vi "SG Main.vi"() -> ()   [LabVIEW 2019]
uses:
  UI Controls/redRoundButton.ctl
  TypeDefs/SG States.ctl
  TypeDefs/SG Data.ctl
  Player/Player.lvclass
  Simon_Engine/Simon_Engine.lvclass
  TextDisplay/TextDisplay Class.lvclass
  Messages/simonMessages/simonMessages.lvclass
  uiControlsMgr/uiControlsMgr.lvclass
  Player/Player.lvclass/Player.ctl
  e5cb8d52-8214-47cd-985f-bfccfb8a6597.vi
  <vilib>/ErrorRing/Error Ring.xnode
panel:
  in  "0008":bool caption="REPETE"
  in  "0007":bool caption="MAIS LONGO"
  in  "0006":T1 caption="PARTIDA"
  in  "0005":u8(slide)=1 caption="HABILIDADE" min=1 max=5 step=1 scale=1.0..4.0
  in  "0001":bool caption="Vermelho"
  in  "0004":bool caption="Amarelo"
  in  "0003":bool caption="Verde"
  in  "0002":bool caption="Azul"
  out "0009":string caption="MOSTRADOR"
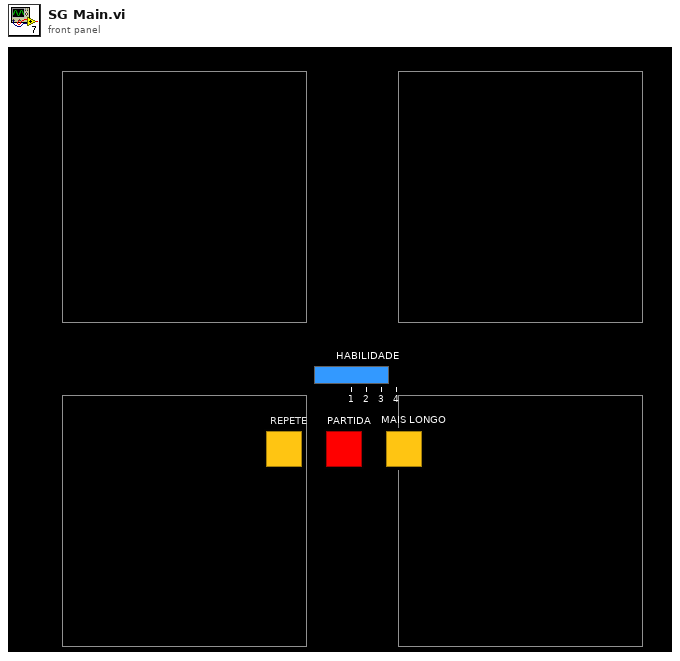
[diagram p1: front panel]
types:
  T1 = typedef "redRoundButton.ctl" = bool
  T2 = typedef "SG Data.ctl" = cluster{"Player":refnum<class "Player.lvclass">, "Engine":refnum<class "Simon_Engine.lvclass">, "TextDisplay":refnum<class "TextDisplay Class.lvclass">, "Messages":refnum<class "simonMessages.lvclass">, "UI Controls Mgr":refnum<class "uiControlsMgr.lvclass">, "High Scores":map{string, i32}, "This VI":refnum<vi>, "LanguageFiles":cluster{"captionsFile":string, "messageFile":string}}
  T3 = typedef "SG States.ctl" = enum16{"Initialize References", "Initialize Classes", "Wait on Event", "Start Game", "Last", "Longest", "Play Game", "Check Move", "Win", "Lost", "HighScores", "Exit"}
  T4 = cluster{"captionsFile":string, "messageFile":string}
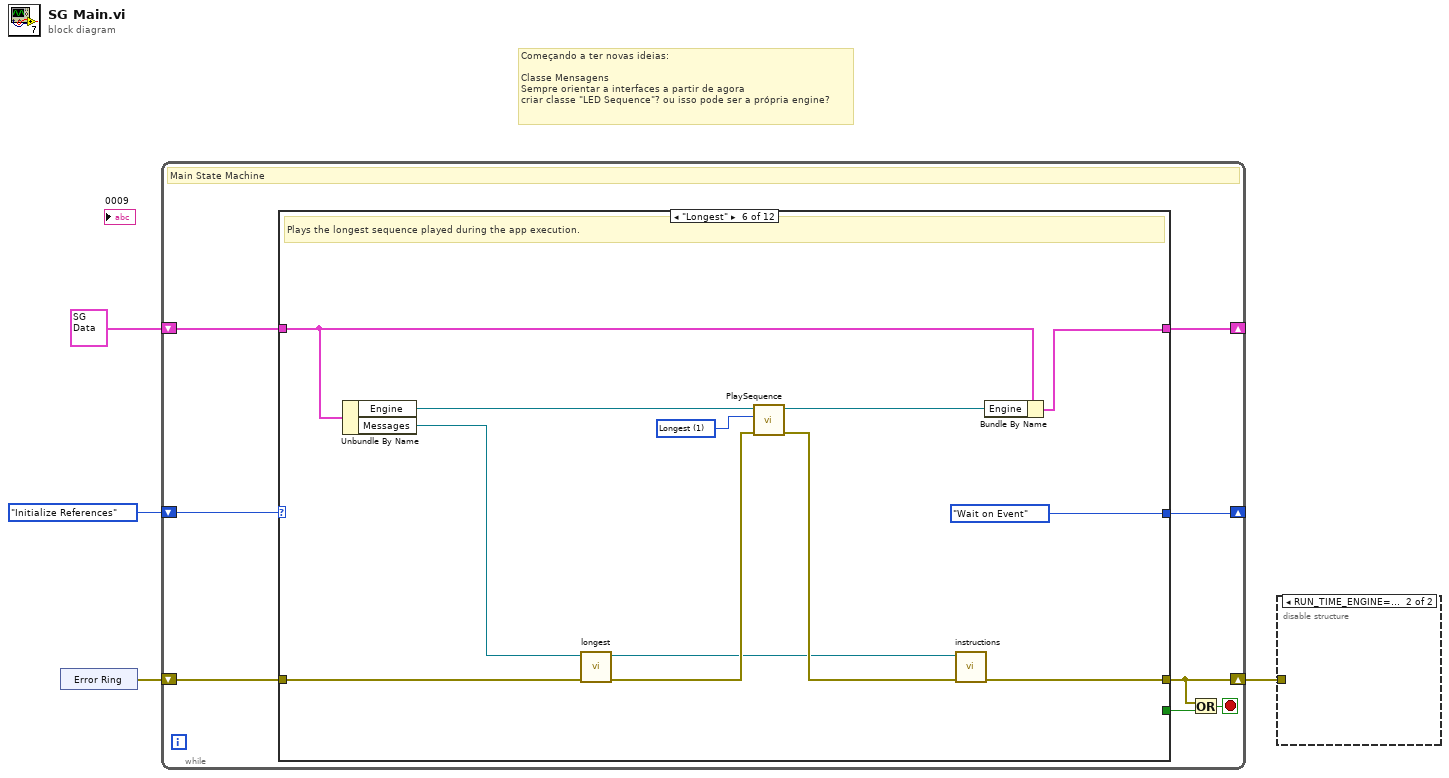
[diagram p0: block diagram]
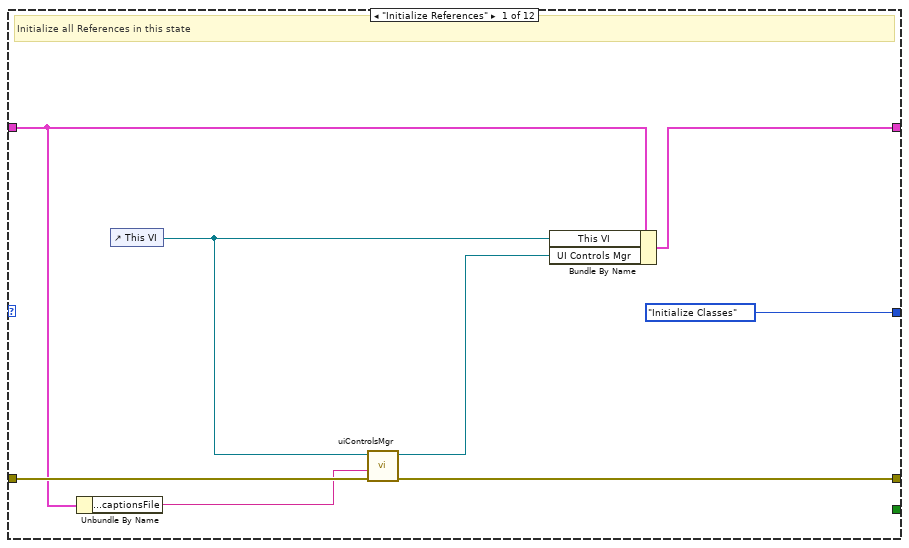
[diagram p2: hidden frame]
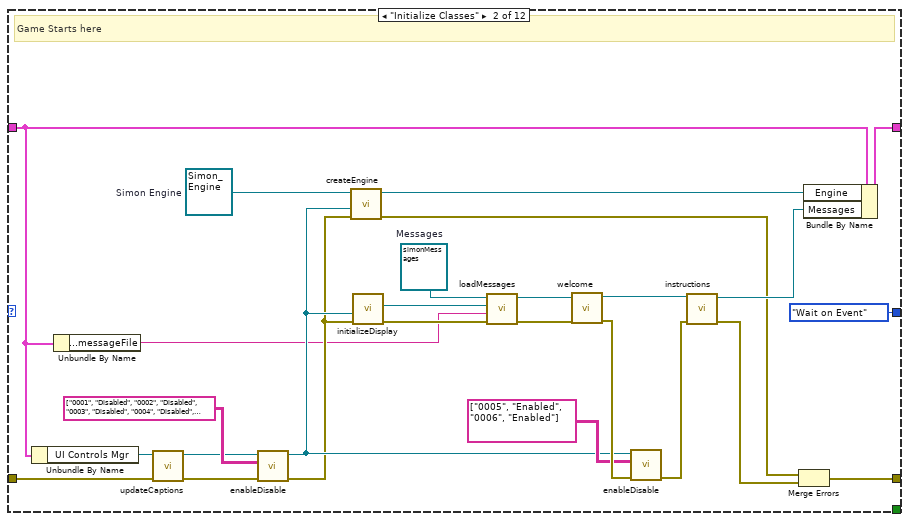
[diagram p3: hidden frame]
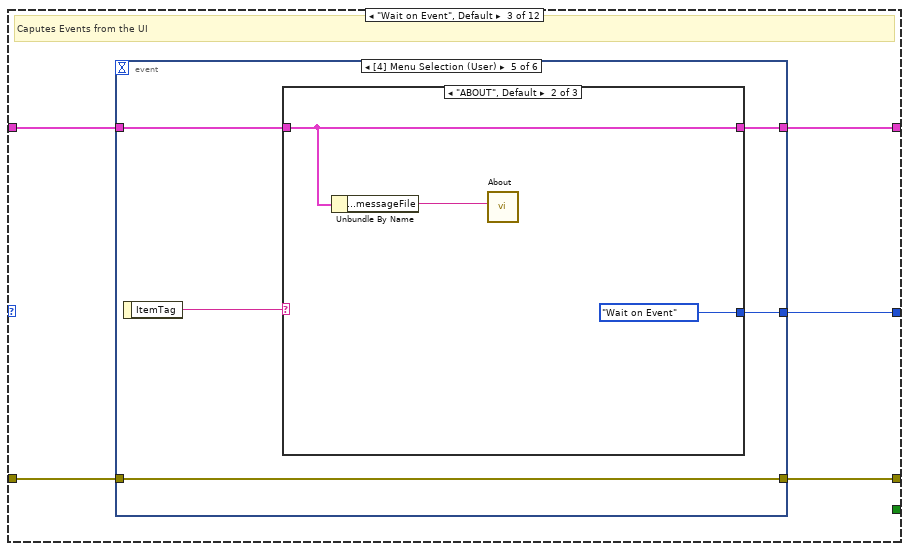
[diagram p4: hidden frame]
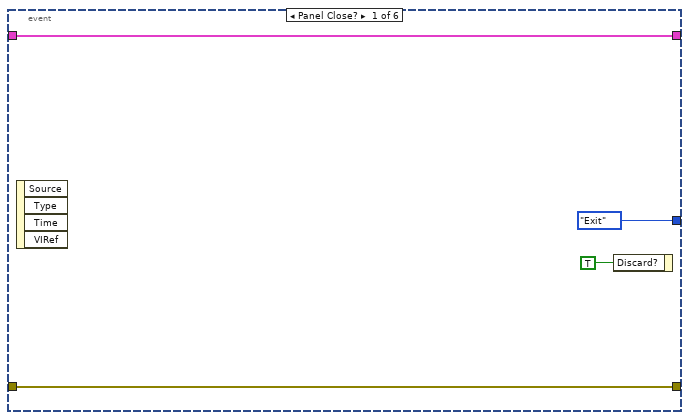
[diagram p5: hidden frame]
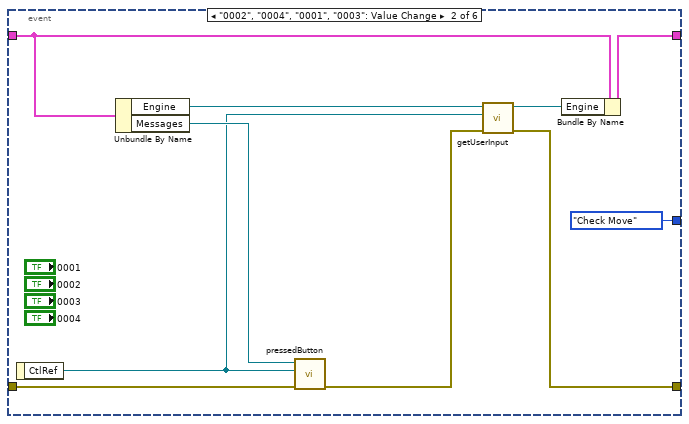
[diagram p6: hidden frame]
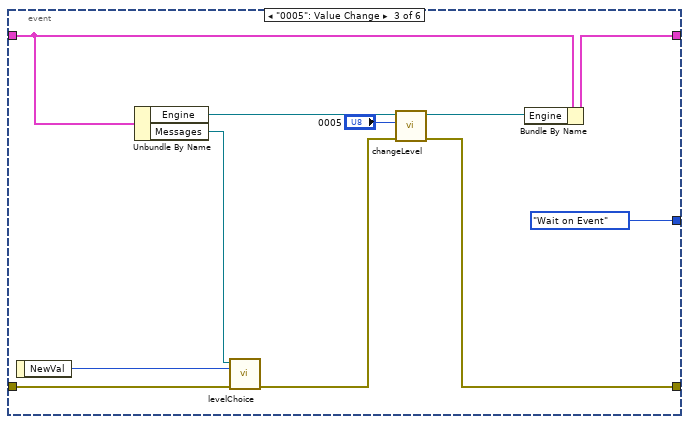
[diagram p7: hidden frame]
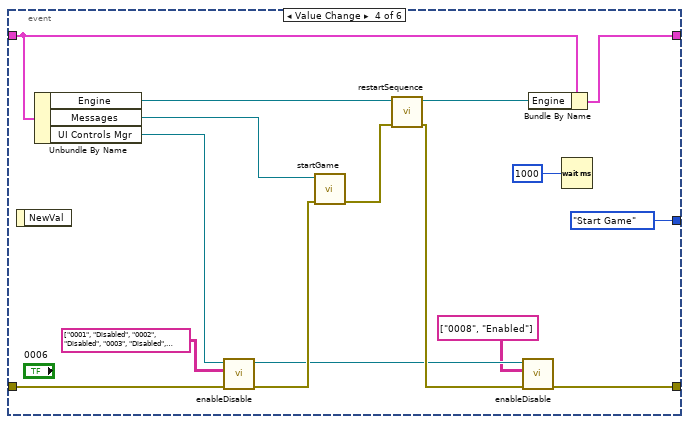
[diagram p8: hidden frame]
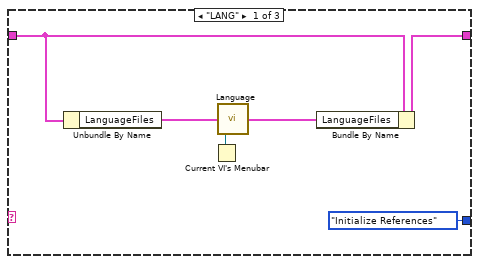
[diagram p9: hidden frame]
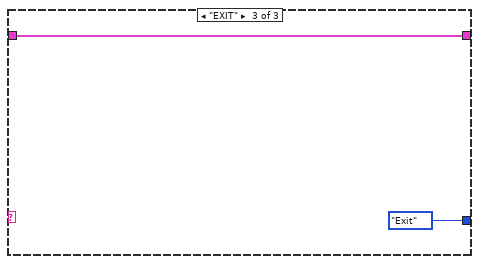
[diagram p10: hidden frame]
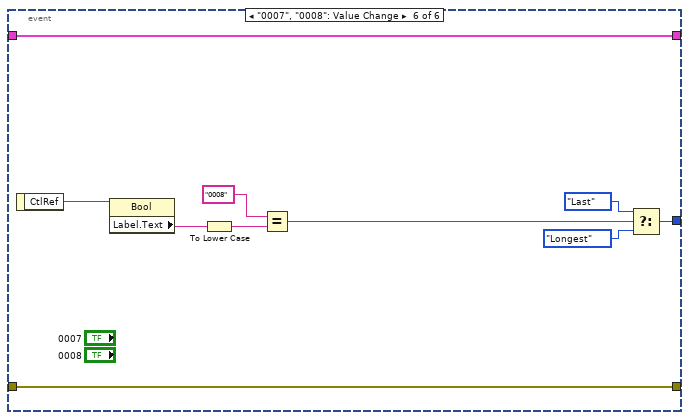
[diagram p11: hidden frame]
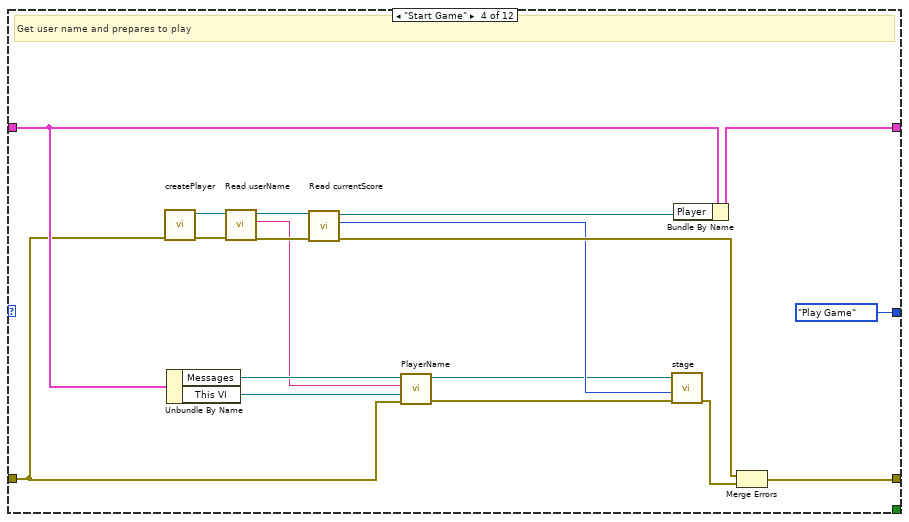
[diagram p12: hidden frame]
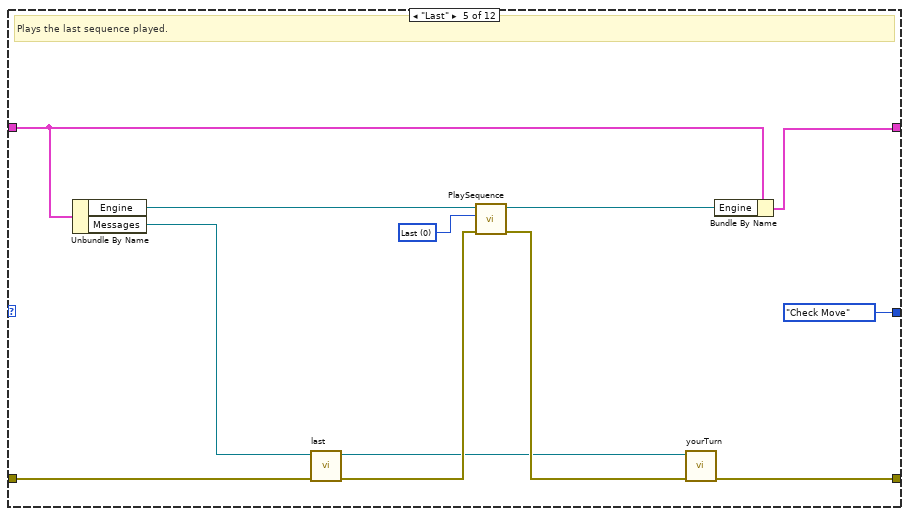
[diagram p13: hidden frame]
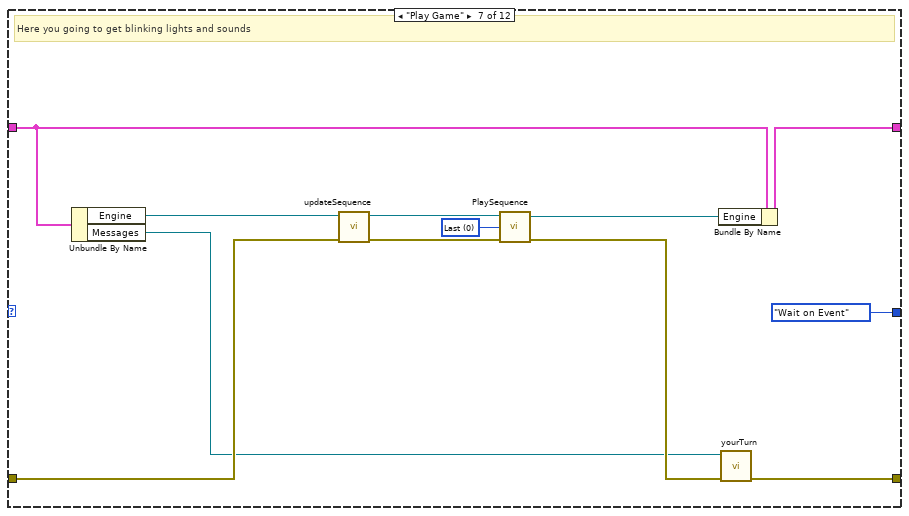
[diagram p14: hidden frame]
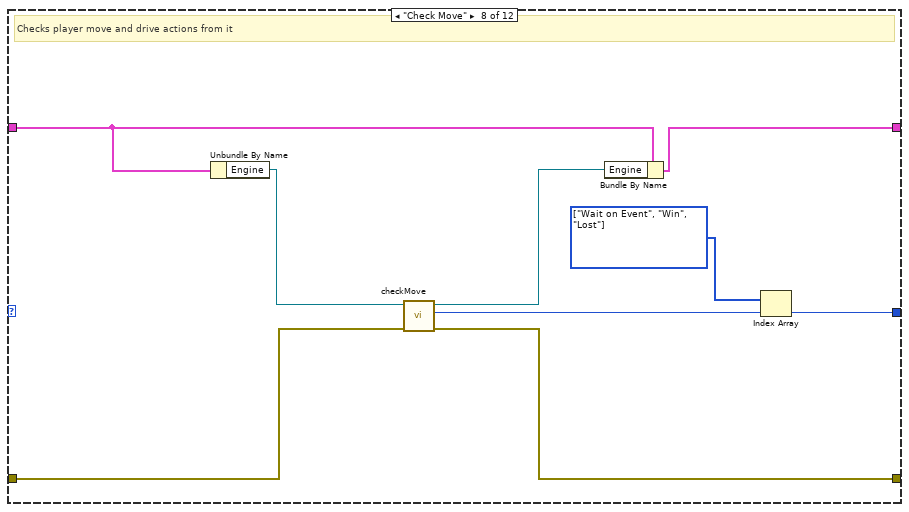
[diagram p15: hidden frame]
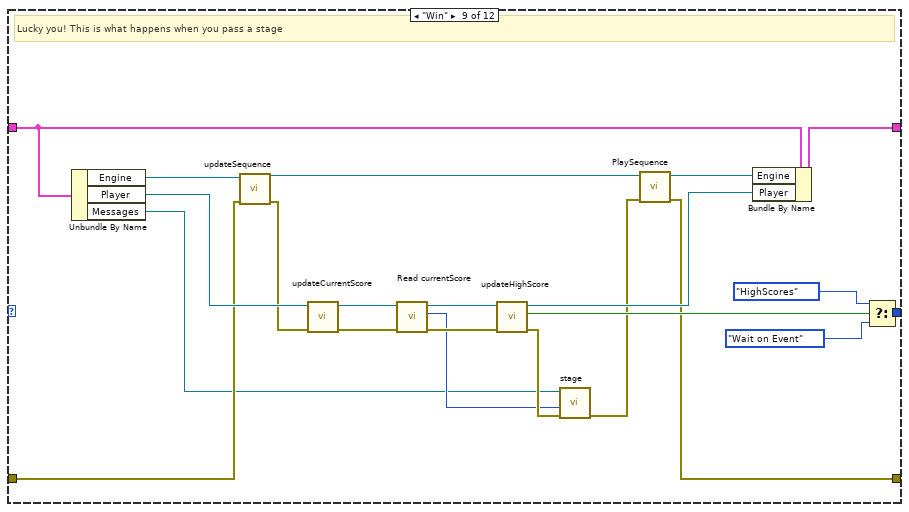
[diagram p16: hidden frame]
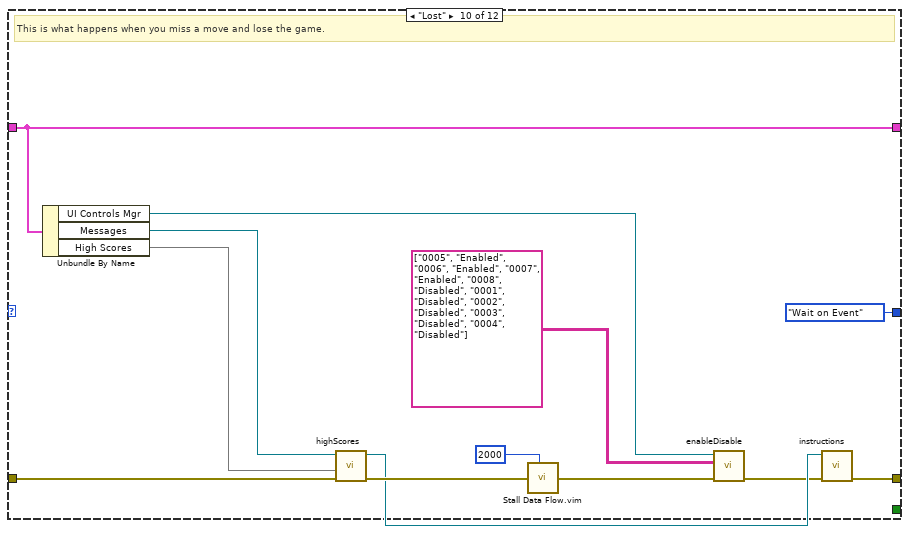
[diagram p17: hidden frame]
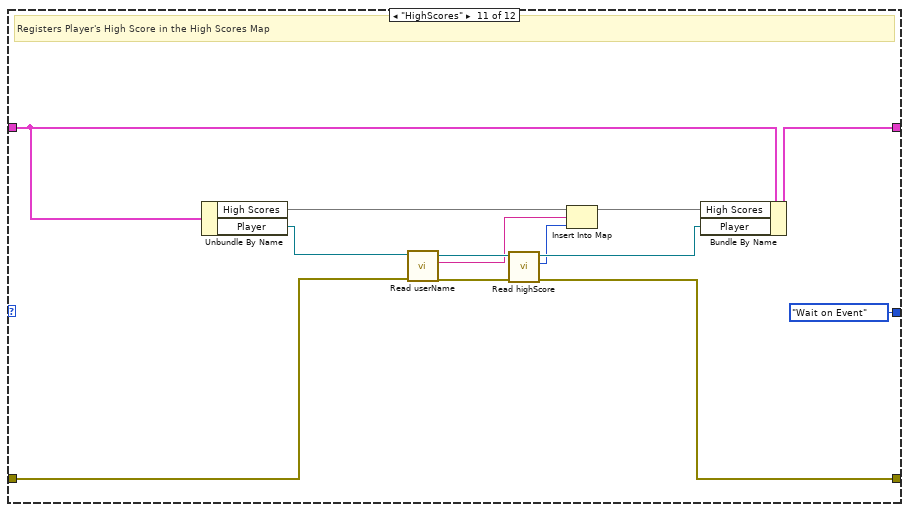
[diagram p18: hidden frame]
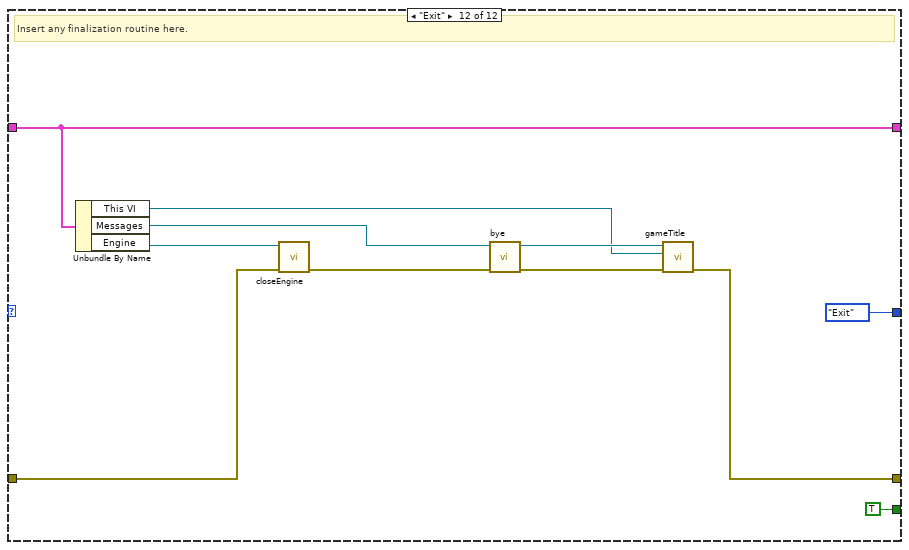
[diagram p19: hidden frame]
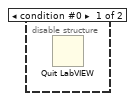
[diagram p20: hidden frame]
diagram:
  # "Começando a ter novas ideias:\n\nClasse Mensagens\nSempre orientar a interfaces a partir de agora\ncriar classe \"LED Sequence\"? ou isso pode ser a própria engine?"
  n1 = xnode "Error Ring"() -> ("error out"=w3:errorcluster)
  n2 = while {
    shift-right: [w11] -> _
    shift-left: T2 {"Player"=refnum, "Engine"=refnum, "TextDisplay"=refnum, "Messages"=refnum, "UI Controls Mgr"=refnum, "High Scores"={}, "This VI"=refnum, "LanguageFiles"={"captionsFile"="captions_english", "messageFile"="messagesEN"}} ("SG Data") -> [w10]
    shift-right: [w8] -> _
    shift-left: SG_States."Initialize References" ("SG States") -> [w12]
    shift-right: [w5] -> w2
    shift-left: w3 -> [w7]
    stop <- w6 stop-if-true
    # "Main State Machine"
    n3 = case shown="\"Longest\"" w12 {
      tunnel: [w20 w46 w49 w130 w143 w155 w172 w181 w202 w215 w228 w238] -> w11
      tunnel: w10 -> [w15 w22 w51 w131 w144 w156 w171 w180 w203 w215 w227 w238]
      tunnel: [_ _ _ _ _ _ _ _ _ _ _ TRUE] -> w9
      tunnel: [SG_States."Initialize Classes" ("SG States") SG_States."Wait on Event" ("SG States") w50 SG_States."Play Game" ("SG States") SG_States."Check Move" ("SG States") SG_States."Wait on Event" ("SG States") SG_States."Wait on Event" ("SG States") w176 w191 SG_States."Wait on Event" ("SG States") SG_States."Wait on Event" ("SG States") SG_States."Exit" ("SG States")] -> w8
      tunnel: w7 -> [w18 w42 w48 w119 w146 w158 w165 w174 w186 w214 w218 w235]
      tunnel: [w17 w24 w47 w128 w138 w150 w163 w173 w185 w209 w217 w233] -> w5
      frame "Initialize References" {
        # "Initialize all References in this state"
        n4 = Unbundle By Name(w15) -> ("LanguageFiles.captionsFile"=w14:string)
        n5 = control-ref of="This VI"() -> (w13:refnum<vi>)
        n6 = call "uiControlsMgr.vi"("error in (no error)"=w18, "Captions File"=w14, "VI reference"=w13) -> ("error out"=w17:errorcluster, "uiControlsMgr out"=w16:refnum<class "uiControlsMgr.lvclass">)  [unwired: 7 in]
        n7 = Bundle By Name(cluster=w15, "This VI"=w13, "UI Controls Mgr"=w16) -> (w20:T2)
      }
      frame "Initialize Classes" {
        w40 = refnum<class "simonMessages.lvclass"> refnum  # Messages
        w43 = refnum<class "Simon_Engine.lvclass"> refnum  # Simon Engine
        # "Game Starts here"
        n8 = Unbundle By Name(w22) -> ("UI Controls Mgr"=w27:refnum<class "uiControlsMgr.lvclass">)
        n9 = Unbundle By Name(w22) -> ("LanguageFiles.messageFile"=w21:string)
        n10 = call "updateCaptions.vi"("error in (no error)"=w42, "uiControlsMgr in"=w27) -> ("error out"=w28:errorcluster, "uiControlsMgr out"=w26:refnum<class "uiControlsMgr.lvclass">)  [unwired: 8 in]
        n11 = call "enableDisable.vi"("error in (no error)"=w28, "Controls - Status"=string[][] [["0001", "Disabled"], ["0002", "Disabled"], ["0003", "Disabled"], ["0004", "Disabled"], ["0005", "Disabled"], ["0006", "Disabled"], ["0007", "Disabled"], ["0008", "Disabled"]], "uiControlsMgr in"=w26) -> ("error out"=w25:errorcluster, "uiControlsMgr out"=w29:refnum<class "uiControlsMgr.lvclass">)  [unwired: 7 in]
        n12 = call-dynamic "createEngine.vi"("error in (no error)"=w25, "uiControlsMgr.lvclass"=w29, "Simon_Engine in"=w43) -> ("error out"=w23:errorcluster, "Simon_Engine out"=w45:refnum<class "Simon_Engine.lvclass">)  [unwired: 7 in]
        n13 = call "initializeDisplay.vi"("error in (no error)"=w25, "uiControlsMgr.lvclass"=w29) -> ("error out"=w39:errorcluster, "TextDisplay Class out"=w36:refnum<class "TextDisplay Class.lvclass">)  [unwired: 8 in]
        n14 = call "loadMessages.vi"("error in (no error)"=w39, "FileName (without extension)"=w21, "TextDisplay"=w36, "simonMessages in"=w40) -> ("error out"=w38:errorcluster, "simonMessages out"=w37:refnum<class "simonMessages.lvclass">)  [unwired: 6 in]
        n15 = call "welcome.vi"("error in (no error)"=w38, "simonMessages in"=w37) -> ("error out"=w33:errorcluster, "simonMessages out"=w35:refnum<class "simonMessages.lvclass">)  [unwired: 8 in]
        n16 = call "enableDisable.vi"("error in (no error)"=w33, "Controls - Status"=string[][] [["0005", "Enabled"], ["0006", "Enabled"]], "uiControlsMgr in"=w29) -> ("error out"=w32:errorcluster)  [unwired: 7 in, 1 out]
        n17 = call "instructions.vi"("error in (no error)"=w32, "simonMessages in"=w35) -> ("error out"=w41:errorcluster, "simonMessages out"=w34:refnum<class "simonMessages.lvclass">)  [unwired: 8 in]
        n18 = Merge Errors(w23, w41) -> (w24:errorcluster)
        n19 = Bundle By Name(cluster=w22, "Engine"=w45, "Messages"=w34) -> (w46:T2)
      }
      frame "Wait on Event", Default {
        # "Caputes Events from the UI"
        n20 = event shown="[4] Menu Selection (User)" {
          selector: _ -> [_ _ _ _ _ _]
          dyn-events: _ -> [_ _ _ _ _ _]
          timeout: _ -> [_ _ _ _ _ _]
          tunnel: w51 -> [w55 w65 w75 w87 w95 w117]
          tunnel: [w55 w63 w76 w91 w94 w117] -> w49
          tunnel: [SG_States."Exit" ("SG States") SG_States."Check Move" ("SG States") SG_States."Wait on Event" ("SG States") SG_States."Start Game" ("SG States") w93 w113] -> w50
          tunnel: w48 -> [w52 w60 w70 w86 w97 w118]
          tunnel: [w52 w59 w69 w84 w97 w118] -> w47
          event Panel Close? {
            n21 = event-data() -> ()  [unwired: 1 in, 4 out]
            n22 = event-data("Discard?"=TRUE) -> ()  [unwired: 1 in, 1 out]
          }
          event "0002", "0004", "0001", "0003": Value Change {
            n23 = event-data() -> ("CtlRef"=w56:refnum<vi>)  [unwired: 1 in]
            n24 = Unbundle By Name(w65) -> ("Engine"=w64:refnum<class "Simon_Engine.lvclass">, "Messages"=w57:refnum<class "simonMessages.lvclass">)
            n25 = call "pressedButton.vi"("error in (no error)"=w60, "Bool Refnum"=w56, "simonMessages in"=w57) -> ("error out"=w58:errorcluster)  [unwired: 7 in, 1 out]
            n26 = call-dynamic "getUserInput.vi"("error in (no error)"=w58, "clickedLEDReference"=w56, "Simon_Engine in"=w64) -> ("error out"=w59:errorcluster, "Simon_Engine out"=w62:refnum<class "Simon_Engine.lvclass">)  [unwired: 7 in]
            n27 = Bundle By Name(cluster=w65, "Engine"=w62) -> (w63:T2)
          }
          event "0005": Value Change {
            n28 = event-data() -> ("NewVal"=w66:u8)  [unwired: 1 in]
            n29 = Unbundle By Name(w75) -> ("Engine"=w74:refnum<class "Simon_Engine.lvclass">, "Messages"=w67:refnum<class "simonMessages.lvclass">)
            n30 = call "levelChoice.vi"("error in (no error)"=w70, "Level Number"=w66, "simonMessages in"=w67) -> ("error out"=w68:errorcluster)  [unwired: 7 in, 1 out]
            n31 = call-dynamic "changeLevel.vi"("error in (no error)"=w68, "Level"="0005", "Simon_Engine in"=w74) -> ("error out"=w69:errorcluster, "Simon_Engine out"=w73:refnum<class "Simon_Engine.lvclass">)  [unwired: 7 in]
            n32 = Bundle By Name(cluster=w75, "Engine"=w73) -> (w76:T2)
          }
          event Value Change {
            n33 = event-data() -> ()  [unwired: 1 in, 1 out]
            n34 = Unbundle By Name(w87) -> ("Engine"=w90:refnum<class "Simon_Engine.lvclass">, "Messages"=w82:refnum<class "simonMessages.lvclass">, "UI Controls Mgr"=w79:refnum<class "uiControlsMgr.lvclass">)
            n35 = call "enableDisable.vi"("error in (no error)"=w86, "Controls - Status"=string[][] [["0001", "Disabled"], ["0002", "Disabled"], ["0003", "Disabled"], ["0004", "Disabled"], ["0005", "Disabled"], ["0006", "Disabled"], ["0007", "Disabled"]], "uiControlsMgr in"=w79) -> ("error out"=w81:errorcluster, "uiControlsMgr out"=w78:refnum<class "uiControlsMgr.lvclass">)  [unwired: 7 in]
            n36 = call "startGame.vi"("error in (no error)"=w81, "simonMessages in"=w82) -> ("error out"=w83:errorcluster)  [unwired: 8 in, 1 out]
            n37 = call-dynamic "restartSequence.vi"("error in (no error)"=w83, "Simon_Engine in"=w90) -> ("error out"=w85:errorcluster, "Simon_Engine out"=w89:refnum<class "Simon_Engine.lvclass">)  [unwired: 8 in]
            n38 = call "enableDisable.vi"("error in (no error)"=w85, "Controls - Status"=string[][] [["0008", "Enabled"]], "uiControlsMgr in"=w78) -> ("error out"=w84:errorcluster)  [unwired: 7 in, 1 out]
            n39 = Bundle By Name(cluster=w87, "Engine"=w89) -> (w91:T2)
            n40 = Wait (ms)(milliseconds to wait=u32 1000) -> ()  [unwired: 1 out]
          }
          event Menu Selection (User) {
            n41 = event-data() -> ("ItemTag"=w96:string)  [unwired: 1 in]
            n42 = case shown="\"ABOUT\", Default" w96 {
              tunnel: w95 -> [w101 w105 w108]
              tunnel: [w99 w105 w108] -> w94
              tunnel: [SG_States."Initialize References" ("SG States") SG_States."Wait on Event" ("SG States") SG_States."Exit" ("SG States")] -> w93
              frame "LANG" {
                n43 = Unbundle By Name(w101) -> ("LanguageFiles"=w100:T4)
                n44 = Current VI's Menubar() -> (w102:refnum<k9>)
                n45 = call "Language.vi"("menu reference"=w102, "LanguageFiles"=w100) -> ("LanguageFiles Out"=w98:T4)  [unwired: 3 in]
                n46 = Bundle By Name(cluster=w101, "LanguageFiles"=w98) -> (w99:T2)
              }
              frame "ABOUT", Default {
                n47 = Unbundle By Name(w105) -> ("LanguageFiles.messageFile"=w104:string)
                n48 = call "About.vi"("FileName (without extension)"=w104) -> ()  [unwired: 11 in]
              }
              frame "EXIT" {
              }
            }
          }
          event "0007", "0008": Value Change {
            n49 = event-data() -> ("CtlRef"=w116:refnum<vi>)  [unwired: 1 in]
            n50 = property class="Bool"(reference=w116) -> ("Label.Text"=w112:string)  [unwired: 1 in, 2 out]
            n51 = To Lower Case(string=w112) -> (all lower case string=w110:string)
            n52 = Equal?(x="0008", y=w110) -> (x = y?=w109:bool)
            n53 = Select(t=SG_States."Last" ("SG States"), s=w109, f=SG_States."Longest" ("SG States")) -> (s? t:f=w113:T3)
          }
        }
      }
      frame "Start Game" {
        # "Get user name and prepares to play"
        n54 = call "createPlayer.vi"("error in (no error)"=w119) -> ("error out"=w132:errorcluster, "Player out"=w135:refnum<class "Player.lvclass">)  [unwired: 9 in]
        n55 = Unbundle By Name(w131) -> ("Messages"=w123:refnum<class "simonMessages.lvclass">, "This VI"=w121:refnum<vi>)
        n56 = call "Read userName.vi"("error in (no error)"=w132, "Player in"=w135) -> ("error out"=w133:errorcluster, "userName"=w120:string, "Player out"=w134:refnum<class "Player.lvclass">)  [unwired: 7 in]
        n57 = call "Read currentScore.vi"("error in (no error)"=w133, "Player in"=w134) -> ("error out"=w127:errorcluster, "currentScore"=w125:u64, "Player out"=w129:refnum<class "Player.lvclass">)  [unwired: 7 in]
        n58 = call "PlayerName.vi"("error in (no error)"=w119, "VI Refnum"=w121, "PlayerName"=w120, "simonMessages in"=w123) -> ("error out"=w124:errorcluster, "simonMessages out"=w122:refnum<class "simonMessages.lvclass">)  [unwired: 6 in]
        n59 = call "stage.vi"("error in (no error)"=w124, "stage number"=w125, "simonMessages in"=w122) -> ("error out"=w126:errorcluster)  [unwired: 7 in, 1 out]
        n60 = Bundle By Name(cluster=w131, "Player"=w129) -> (w130:T2)
        n61 = Merge Errors(w127, w126) -> (w128:errorcluster)
      }
      frame "Last" {
        w141 = u8 0 items=["Last", "Longest"] ("Sequence")
        # "Plays the last sequence played."
        n62 = Unbundle By Name(w144) -> ("Engine"=w147:refnum<class "Simon_Engine.lvclass">, "Messages"=w139:refnum<class "simonMessages.lvclass">)
        n63 = call "last.vi"("error in (no error)"=w146, "simonMessages in"=w139) -> ("error out"=w140:errorcluster, "simonMessages out"=w137:refnum<class "simonMessages.lvclass">)  [unwired: 8 in]
        n64 = call-dynamic "PlaySequence.vi"("error in (no error)"=w140, "Sequence"=w141, "Simon_Engine in"=w147) -> ("error out"=w145:errorcluster, "Simon_Engine out"=w148:refnum<class "Simon_Engine.lvclass">)  [unwired: 7 in]
        n65 = call "yourTurn.vi"("error in (no error)"=w145, "simonMessages in"=w137) -> ("error out"=w138:errorcluster)  [unwired: 8 in, 1 out]
        n66 = Bundle By Name(cluster=w144, "Engine"=w148) -> (w143:T2)
      }
      frame "Longest" {
        w153 = u8 1 items=["Last", "Longest"] ("Sequence")
        # "Plays the longest sequence played during the app execution."
        n67 = Unbundle By Name(w156) -> ("Engine"=w159:refnum<class "Simon_Engine.lvclass">, "Messages"=w151:refnum<class "simonMessages.lvclass">)
        n68 = call "longest.vi"("error in (no error)"=w158, "simonMessages in"=w151) -> ("error out"=w152:errorcluster, "simonMessages out"=w149:refnum<class "simonMessages.lvclass">)  [unwired: 8 in]
        n69 = call-dynamic "PlaySequence.vi"("error in (no error)"=w152, "Sequence"=w153, "Simon_Engine in"=w159) -> ("error out"=w157:errorcluster, "Simon_Engine out"=w160:refnum<class "Simon_Engine.lvclass">)  [unwired: 7 in]
        n70 = call "instructions.vi"("error in (no error)"=w157, "simonMessages in"=w149) -> ("error out"=w150:errorcluster)  [unwired: 8 in, 1 out]
        n71 = Bundle By Name(cluster=w156, "Engine"=w160) -> (w155:T2)
      }
      frame "Play Game" {
        w161 = u8 0 items=["Last", "Longest"] ("Sequence")
        # "Here you going to get blinking lights and sounds"
        n72 = Unbundle By Name(w171) -> ("Engine"=w170:refnum<class "Simon_Engine.lvclass">, "Messages"=w162:refnum<class "simonMessages.lvclass">)
        n73 = call-dynamic "updateSequence.vi"("error in (no error)"=w165, "Simon_Engine in"=w170) -> ("error out"=w168:errorcluster, "Simon_Engine out"=w169:refnum<class "Simon_Engine.lvclass">)  [unwired: 8 in]
        n74 = call-dynamic "PlaySequence.vi"("error in (no error)"=w168, "Sequence"=w161, "Simon_Engine in"=w169) -> ("error out"=w164:errorcluster, "Simon_Engine out"=w167:refnum<class "Simon_Engine.lvclass">)  [unwired: 7 in]
        n75 = Bundle By Name(cluster=w171, "Engine"=w167) -> (w172:T2)
        n76 = call "yourTurn.vi"("error in (no error)"=w164, "simonMessages in"=w162) -> ("error out"=w163:errorcluster)  [unwired: 8 in, 1 out]
      }
      frame "Check Move" {
        w177 = T3[] [enum."Wait on Event", enum."Win", enum."Lost"] items=["Initialize References", "Initialize Classes", "Wait on Event", "Start Game", "Last", "Longest", "Play Game", "Check Move", "Win", "Lost", "HighScores", "Exit"] ("Array")
        # "Checks player move and drive actions from it"
        n77 = Unbundle By Name(w180) -> ("Engine"=w179:refnum<class "Simon_Engine.lvclass">)
        n78 = call-dynamic "checkMove.vi"("error in (no error)"=w174, "Simon_Engine in"=w179) -> ("error out"=w173:errorcluster, "MachStatus"=w175:i16, "Simon_Engine out"=w178:refnum<class "Simon_Engine.lvclass">)  [unwired: 7 in]
        n79 = Bundle By Name(cluster=w180, "Engine"=w178) -> (w181:T2)
        n80 = Index Array(array=w177, index=w175) -> (element=w176:T3)
      }
      frame "Win" {
        # "Lucky you! This is what happens when you pass a stage"
        n81 = Unbundle By Name(w203) -> ("Engine"=w201:refnum<class "Simon_Engine.lvclass">, "Player"=w196:refnum<class "Player.lvclass">, "Messages"=w182:refnum<class "simonMessages.lvclass">)
        n82 = call-dynamic "updateSequence.vi"("error in (no error)"=w186, "Simon_Engine in"=w201) -> ("error out"=w190:errorcluster, "Simon_Engine out"=w200:refnum<class "Simon_Engine.lvclass">)  [unwired: 8 in]
        n83 = call "updateCurrentScore.vi"("error in (no error)"=w190, "Player in"=w196) -> ("error out"=w189:errorcluster, "Player out"=w195:refnum<class "Player.lvclass">)  [unwired: 8 in]
        n84 = call "Read currentScore.vi"("error in (no error)"=w189, "Player in"=w195) -> ("error out"=w188:errorcluster, "currentScore"=w183:u64, "Player out"=w198:refnum<class "Player.lvclass">)  [unwired: 7 in]
        n85 = call "updateHighScore.vi"("error in (no error)"=w188, "Player in"=w198) -> ("error out"=w187:errorcluster, "High Score Updated?"=w192:bool, "Player out"=w197:refnum<class "Player.lvclass">)  [unwired: 7 in]
        n86 = call "stage.vi"("error in (no error)"=w187, "stage number"=w183, "simonMessages in"=w182) -> ("error out"=w184:errorcluster)  [unwired: 7 in, 1 out]
        n87 = call-dynamic "PlaySequence.vi"("error in (no error)"=w184, "Simon_Engine in"=w200) -> ("error out"=w185:errorcluster, "Simon_Engine out"=w199:refnum<class "Simon_Engine.lvclass">)  [unwired: 8 in]
        n88 = Bundle By Name(cluster=w203, "Engine"=w199, "Player"=w197) -> (w202:T2)
        n89 = Select(t=SG_States."HighScores" ("SG States"), s=w192, f=SG_States."Wait on Event" ("SG States")) -> (s? t:f=w191:T3)
      }
      frame "Lost" {
        # "This is what happens when you miss a move and lose the game."
        n90 = Unbundle By Name(w215) -> ("UI Controls Mgr"=w205:refnum<class "uiControlsMgr.lvclass">, "Messages"=w208:refnum<class "simonMessages.lvclass">, "High Scores"=w212:map{string, i32})
        n91 = call "highScores.vi"("error in (no error)"=w214, "High Scores"=w212, "simonMessages in"=w208) -> ("error out"=w213:errorcluster, "simonMessages out"=w207:refnum<class "simonMessages.lvclass">)  [unwired: 7 in]
        n92 = call "Stall Data Flow.vim"("value in"=w213, "milliseconds to wait"=u32 2000) -> ("value out"=w211:errorcluster)  [unwired: 1 out]
        n93 = call "enableDisable.vi"("error in (no error)"=w211, "Controls - Status"=string[][] [["0005", "Enabled"], ["0006", "Enabled"], ["0007", "Enabled"], ["0008", "Disabled"], ["0001", "Disabled"], ["0002", "Disabled"], ["0003", "Disabled"], ["0004", "Disabled"]], "uiControlsMgr in"=w205) -> ("error out"=w206:errorcluster)  [unwired: 7 in, 1 out]
        n94 = call "instructions.vi"("error in (no error)"=w206, "simonMessages in"=w207) -> ("error out"=w209:errorcluster)  [unwired: 8 in, 1 out]
      }
      frame "HighScores" {
        # "Registers Player's High Score in the High Scores Map"
        n95 = Unbundle By Name(w227) -> ("High Scores"=w220:map{string, i32}, "Player"=w226:refnum<class "Player.lvclass">)
        n96 = call "Read userName.vi"("error in (no error)"=w218, "Player in"=w226) -> ("error out"=w224:errorcluster, "userName"=w222:string, "Player out"=w225:refnum<class "Player.lvclass">)  [unwired: 7 in]
        n97 = call "Read highScore.vi"("error in (no error)"=w224, "Player in"=w225) -> ("error out"=w217:errorcluster, "highScore"=w221:u64, "Player out"=w223:refnum<class "Player.lvclass">)  [unwired: 7 in]
        n98 = Insert Into Map(map in=w220, key=w222, value=w221) -> (map out=w219:map{string, i32})  [unwired: 2 out]
        n99 = Bundle By Name(cluster=w227, "High Scores"=w219, "Player"=w223) -> (w228:T2)
      }
      frame "Exit" {
        # "Insert any finalization routine here."
        n100 = Unbundle By Name(w238) -> ("This VI"=w230:refnum<vi>, "Messages"=w234:refnum<class "simonMessages.lvclass">, "Engine"=w237:refnum<class "Simon_Engine.lvclass">)
        n101 = call-dynamic "closeEngine.vi"("error in (no error)"=w235, "Simon_Engine in"=w237) -> ("error out"=w236:errorcluster)  [unwired: 8 in, 1 out]
        n102 = call "bye.vi"("error in (no error)"=w236, "simonMessages in"=w234) -> ("error out"=w231:errorcluster, "simonMessages out"=w232:refnum<class "simonMessages.lvclass">)  [unwired: 8 in]
        n103 = call "gameTitle.vi"("error in (no error)"=w231, "VI Refnum"=w230, "simonMessages in"=w232) -> ("error out"=w233:errorcluster)  [unwired: 7 in, 1 out]
      }
    }
    n104 = Or(x=w5, y=w9) -> (x .or. y?=w6:bool)
  }
  n105 = disable-structure shown="RUN_TIME_ENGINE==False, Default" {
    disable-tunnel: w2 -> [_ _]
    frame condition #0 {
      n106 = Quit LabVIEW() -> ()  [unwired: 1 in]
    }
    frame condition #1 (active) {
    }
  }
